vi "Teleop.vi"(10 "Match Info":T1={"Autonomous Elapsed Seconds"=0.0, "TeleOp Elapsed Seconds"=0.0, "Disabled Elapsed Seconds"=0.0, "Visited Autonomous"=FALSE, "Visited TeleOp"=FALSE, "Visited Disabled"=FALSE, "Autonomous Settings"={"Autonomous Style"=enum."Independent", "VI Refnum"=refnum}}, 11 "Call Context":T2) -> ()   [LabVIEW 2019]
doc: "This VI is called for each TeleOp packet received from the DS where the robot is not disabled. It is often used to read from the joysticks and update I/O or to update setpoints for timed control loops. It should complete and return within 20 milliseconds or it may miss DS packets."
uses:
  <vilib>/Rock Robotics/WPI/DriverStation/WPI_DriverStationDerivedRobotMode.ctl
  <vilib>/Rock Robotics/WPI/DriverStation/WPI_DriverStationMatch Info.ctl
  <vilib>/Rock Robotics/WPI/Utilities/WPI_GetSetVariantRefNum.vi
  <vilib>/Rock Robotics/Network Tables/NT Read Number.vi
  Robot Global Data.vi
  <vilib>/Rock Robotics/Network Tables/NT Write Number.vi
panel:
  # "Click here to set min"
  # "Click here to set max"
  # "Click here to set min"
  # "Click here to set max"
  # "Click here to set min"
  # "Click here to set max"
  # "Click here to set min"
  # "Click here to set max"
  # "Click here to set min"
  # "Click here to set max"
  # "Click here to set min"
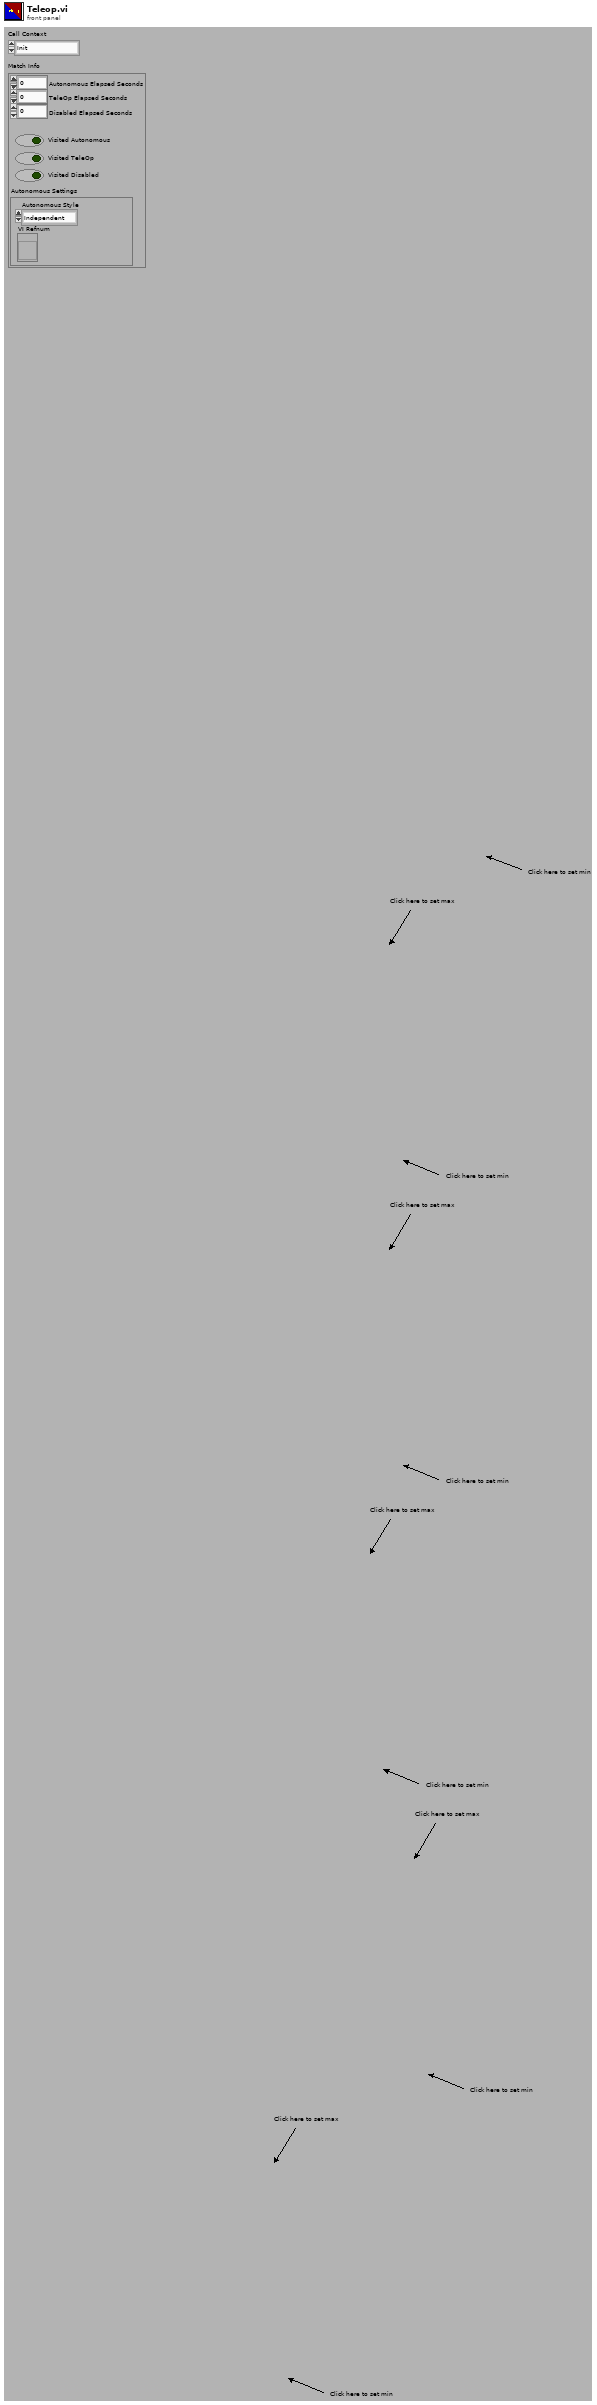
[diagram p1: front panel]
types:
  T1 = typedef "WPI_DriverStationMatch Info.ctl" = cluster{"Autonomous Elapsed Seconds":dbl, "TeleOp Elapsed Seconds":dbl, "Disabled Elapsed Seconds":dbl, "Visited Autonomous":bool, "Visited TeleOp":bool, "Visited Disabled":bool, "Autonomous Settings":cluster{"Autonomous Style":enum16{"Iterative", "Independent"}, "VI Refnum":refnum<vi>}}
  T2 = typedef "WPI_DriverStationDerivedRobotMode.ctl" = enum16{"Init", "Execute", "Stop"}
  T3 = typedef "WPI_MotorControlDeviceRef.ctl" = cluster{"DeviceStatus":errorcluster, "Type":T4, "PWM":cluster{"PWM Channel":T5, "DeadBand":T6}, "CAN":cluster{"Device Number":u8, "SetOutput VI Ref":variant, "GetOutput VI Ref":variant, "Enable VI Ref":variant, "Disable VI Ref":variant, "Data":variant}, "Invert":bool, "DIO PWM":cluster{"PWM \"Enable\" Channel":T5, "DIOChannel":T7, "PWM Rate":dbl}}
  T4 = typedef "WPI_MotorControlType.ctl" = enum16{"PWM", "CAN", "DIO PWM"}
  T5 = typedef "FPGA_DIOPWMChannel.ctl" = enum8{"PWM 0", "PWM 1", "PWM 2", "PWM 3", "PWM 4", "PWM 5", "PWM 6", "PWM 7", "PWM 8", "PWM 9", "PWM MXP 0", "PWM MXP 1", "PWM MXP 2", "PWM MXP 3", "PWM MXP 4", "PWM MXP 5", "PWM MXP 6", "PWM MXP 7", "PWM MXP 8", "PWM MXP 9", "Invalid"}
  T6 = typedef "WPI_PWMDeadband.ctl" = cluster{"Name":string, "maxPositivePwm":i32, "minPositivePwm":i32, "centerPwm":i32, "maxNegativePwm":i32, "minNegativePwm":i32, "angularRange":u16}
  T7 = typedef "FPGA_DIOChannel.ctl" = enum8{"DIO 0", "DIO 1", "DIO 2", "DIO 3", "DIO 4", "DIO 5", "DIO 6", "DIO 7", "DIO 8", "DIO 9", "DIO MXP 0", "DIO MXP 1", "DIO MXP 2", "DIO MXP 3", "DIO MXP 4", "DIO MXP 5", "DIO MXP 6", "DIO MXP 7", "DIO MXP 8", "DIO MXP 9", "DIO MXP 10", "DIO MXP 11", "DIO MXP 12", "DIO MXP 13", "DIO MXP 14", "DIO MXP 15", "SPI Port CS1", "SPI Port CS2", "SPI Port CS3", "SPI Port MISO", "SPI Port MOSI", "Invalid"}
  T8 = typedef "WPI_JoystickDevRef.ctl" = cluster{"Device":T9}
  T9 = typedef "WPI_JoystickDeviceEnum.ctl" = enum16{"USB 0", "USB 1", "USB 2", "USB 3", "USB 4", "USB 5"}
  T10 = typedef "WPI_RobotDriveDevRef.ctl" = cluster{"DevStatus":errorcluster, "Motors[]":T3[], "Square Inputs":bool, "Max Output":dbl}
  T11 = cluster{"JoystickDevRef":T8, "RobotDriveDevRef":T10}
  T12 = typedef "WPI_ServoDeviceRef.ctl" = cluster{"DeviceStatus":errorcluster, "PWM Channel":T5, "DeadBand":T6}
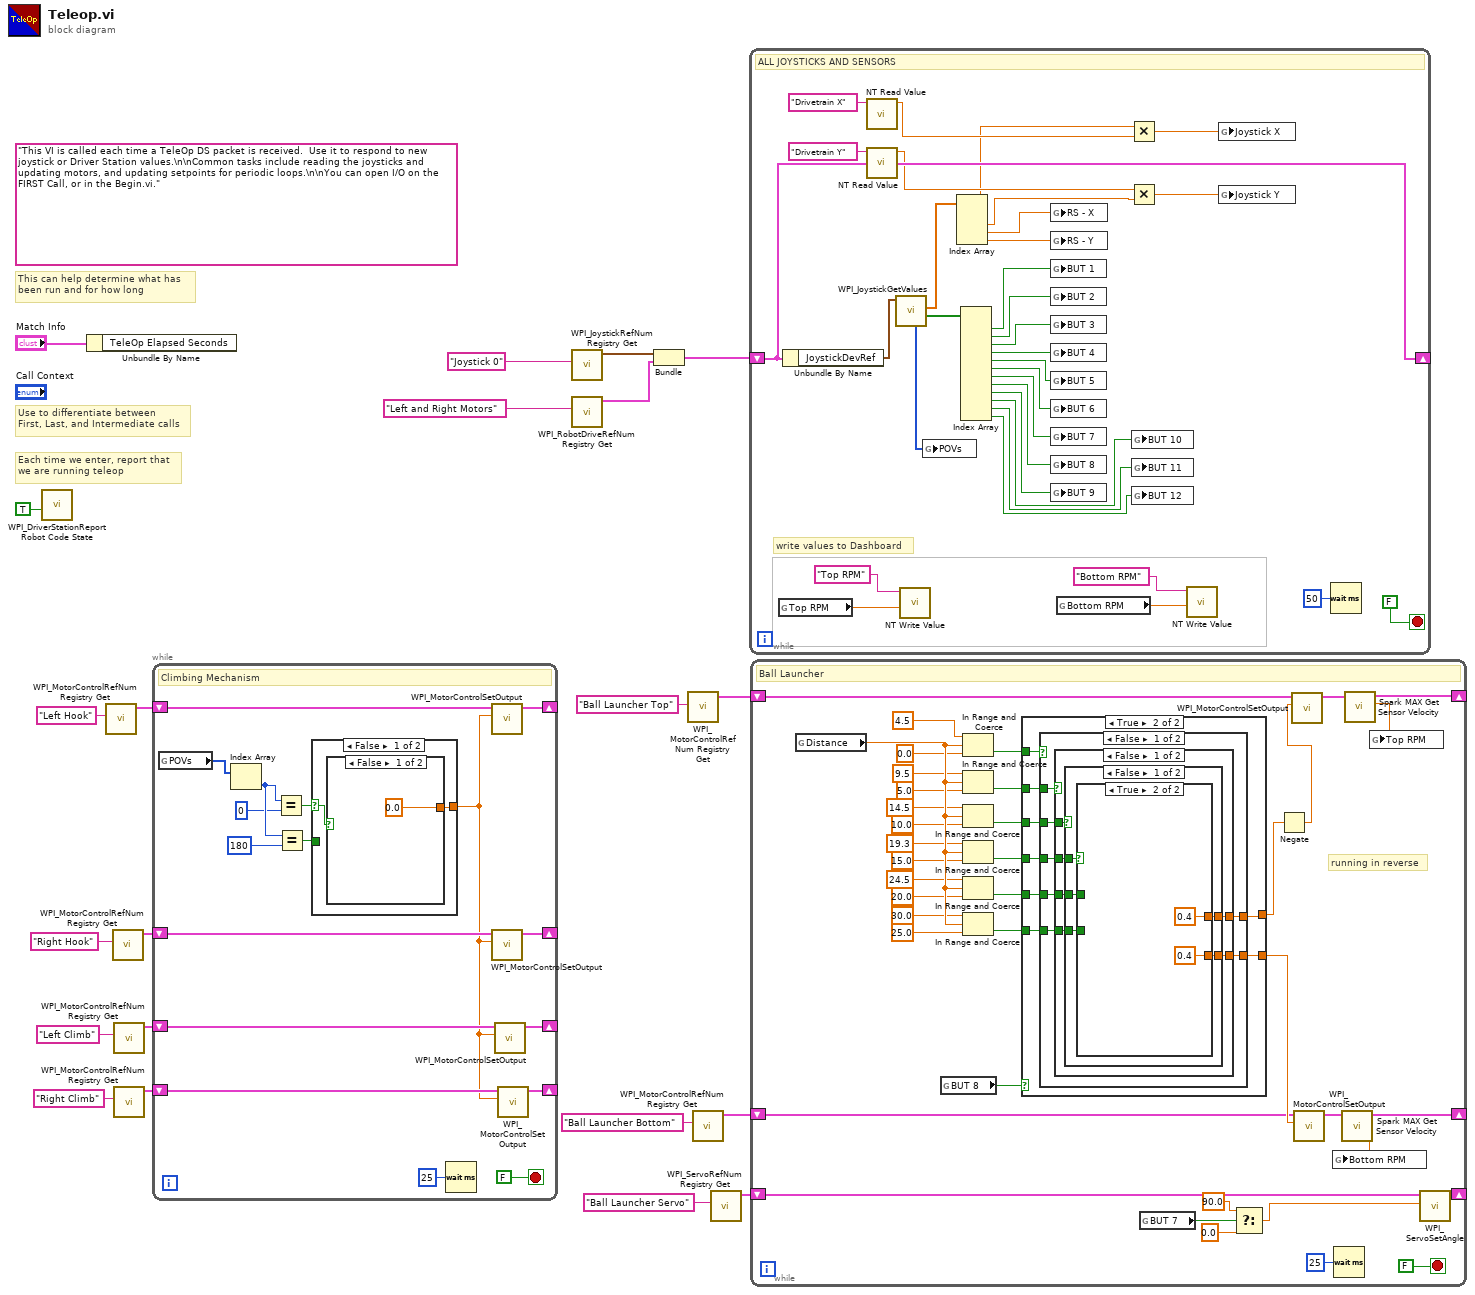
[diagram p0: block diagram]
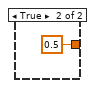
[diagram p2: hidden frame]
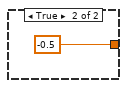
[diagram p3: hidden frame]
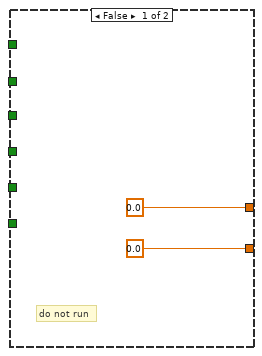
[diagram p4: hidden frame]
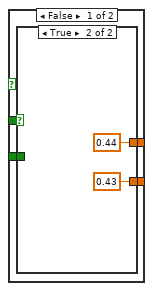
[diagram p5: hidden frame]
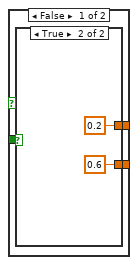
[diagram p6: hidden frame]
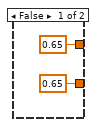
[diagram p7: hidden frame]
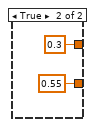
[diagram p8: hidden frame]
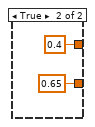
[diagram p9: hidden frame]
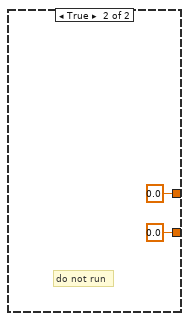
[diagram p10: hidden frame]
diagram:
  (unwired) "This VI is called each time a TeleOp DS packet is received.  Use it to respond to new joystick or Driver Station values.\n\nCommon tasks include reading the joysticks and updating motors, and updating setpoints for periodic loops.\n\nYou can open I/O on the FIRST Call, or in the Begin.vi."
  # "Each time we enter, report that\nwe are running teleop"
  # "Use to differentiate between\nFirst, Last, and Intermediate calls"
  # "This can help determine what has\nbeen run and for how long"
  n1 = call <vilib>:"WPI_DriverStationReport Robot Code State.vi"("TeleOp"=TRUE ("Autonomous")) -> ()  [unwired: 10 in, 1 out]
  n2 = Unbundle By Name("Match Info") -> ()  [unwired: 1 out]
  n3 = call <vilib>:"WPI_MotorControlRefNum Registry Get.vi"("refnum name"="Left Hook") -> ("MotorControlDevRef"=w10:T3)  [unwired: 9 in, 1 out]
  n4 = call <vilib>:"WPI_MotorControlRefNum Registry Get.vi"("refnum name"="Right Hook") -> ("MotorControlDevRef"=w7:T3)  [unwired: 9 in, 1 out]
  n5 = call <vilib>:"WPI_MotorControlRefNum Registry Get.vi"("refnum name"="Left Climb") -> ("MotorControlDevRef"=w3:T3)  [unwired: 9 in, 1 out]
  n6 = call <vilib>:"WPI_MotorControlRefNum Registry Get.vi"("refnum name"="Right Climb") -> ("MotorControlDevRef"=w6:T3)  [unwired: 9 in, 1 out]
  n7 = while {
    shift-right: [w36] -> _
    shift-left: w10 -> [w35]
    shift-right: [w34] -> _
    shift-left: w7 -> [w33]
    shift-right: [w25] -> _
    shift-left: w6 -> [w26]
    shift-right: [w23] -> _
    shift-left: w3 -> [w24]
    stop <- FALSE stop-if-true
    # "Climbing Mechanism"
    n8 = global read "Robot Global Data.vi" "POVs"() -> (w31:i16[])
    n9 = Index Array(array=w31) -> (element=w29:i16)  [unwired: 1 in]
    n10 = Equal?(x=w29, y=i16 0) -> (x = y?=w32:bool)
    n11 = Equal?(x=w29, y=i16 180) -> (x = y?=w30:bool)
    n12 = case shown="False" w32 {
      selector: w32 -> [w39 _]
      tunnel: w30 -> [_ _]
      tunnel: [w40 -0.5 ("Output")] -> w22
      frame False {
        n13 = case shown="False" w39 {
          tunnel: [0.0 ("Output") 0.5 ("Output")] -> w40
          frame False {
          }
          frame True {
          }
        }
      }
      frame True {
      }
    }
    n14 = Wait (ms)(milliseconds to wait=u32 25) -> ()  [unwired: 1 out]
    n15 = call <vilib>:"WPI_MotorControlSetOutput.vi"("Output"=w22, "MotorControlDevRef"=w35) -> ("MotorControlDevRef"=w36:T3)  [unwired: 7 in, 2 out]
    n16 = call <vilib>:"WPI_MotorControlSetOutput.vi"("Output"=w22, "MotorControlDevRef"=w33) -> ("MotorControlDevRef"=w34:T3)  [unwired: 7 in, 2 out]
    n17 = call <vilib>:"WPI_MotorControlSetOutput.vi"("Output"=w22, "MotorControlDevRef"=w24) -> ("MotorControlDevRef"=w23:T3)  [unwired: 7 in, 2 out]
    n18 = call <vilib>:"WPI_MotorControlSetOutput.vi"("Output"=w22, "MotorControlDevRef"=w26) -> ("MotorControlDevRef"=w25:T3)  [unwired: 7 in, 2 out]
  }
  n19 = call <vilib>:"WPI_JoystickRefNum Registry Get.vi"("refnum name"="Joystick 0") -> ("JoystickDevRef"=w17:T8)  [unwired: 1 in, 9 out]
  n20 = call <vilib>:"WPI_RobotDriveRefNum Registry Get.vi"("refnum name"="Left and Right Motors") -> ("RobotDriveDevRef"=w16:T10)  [unwired: 1 in, 9 out]
  n21 = Bundle("JoystickDevRef"=w17, "RobotDriveDevRef"=w16) -> (w15:T11)  [unwired: 1 out]
  n22 = call <vilib>:"WPI_MotorControlRefNum Registry Get.vi"("refnum name"="Ball Launcher Top") -> ("MotorControlDevRef"=w11:T3)  [unwired: 9 in, 1 out]
  n23 = call <vilib>:"WPI_MotorControlRefNum Registry Get.vi"("refnum name"="Ball Launcher Bottom") -> ("MotorControlDevRef"=w13:T3)  [unwired: 9 in, 1 out]
  n24 = call <vilib>:"WPI_ServoRefNum Registry Get.vi"("refnum name"="Ball Launcher Servo") -> ("ServoDeviceRef"=w1:T12)  [unwired: 9 in, 1 out]
  n25 = while {
    shift-right: [w61] -> _
    shift-left: w15 -> [w61]
    stop <- FALSE stop-if-true
    # "write values to Dashboard"
    # "ALL JOYSTICKS AND SENSORS"
    n26 = global read "Robot Global Data.vi" "Top RPM"() -> (w55:dbl)
    n27 = Unbundle By Name(w61) -> ("JoystickDevRef"=w75:T8)
    n28 = call-poly <vilib>:"NT Read Value.vi"("Name"="Drivetrain X") -> ("Numeric"=w49:dbl)  [unwired: 9 in, 1 out]
    n29 = call-poly <vilib>:"NT Read Value.vi"("Name"="Drivetrain Y") -> ("Numeric"=w50:dbl)  [unwired: 9 in, 1 out]
    n30 = call <vilib>:"WPI_JoystickGetValues.vi"("JoystickDevRef"=w75) -> ("Buttons"=w74:bool[], "Axes"=w60:dbl[], "POVs"=w44:i16[])  [unwired: 6 in, 2 out]
    n31 = call-poly <vilib>:"NT Write Value.vi"("Numeric"=w55, "Name"="Top RPM") -> ()  [unwired: 9 in, 1 out]
    n32 = global write "Robot Global Data.vi" "POVs"(w44) -> ()
    n33 = Index Array(array=w60) -> (element #1=w46:dbl, element #2=w45:dbl, element #3=w47:dbl, element #4=w58:dbl)  [unwired: 4 in]
    n34 = Index Array(array=w74) -> (element #1=w73:bool, element #2=w72:bool, element #3=w71:bool, element #4=w70:bool, element #5=w69:bool, element #6=w68:bool, element #7=w67:bool, element #8=w66:bool, element #9=w65:bool, element #10=w64:bool, element #11=w63:bool, element #12=w62:bool)  [unwired: 12 in]
    n35 = global write "Robot Global Data.vi" "RS - X"(w47) -> ()
    n36 = global write "Robot Global Data.vi" "RS - Y"(w58) -> ()
    n37 = global write "Robot Global Data.vi" "BUT 1"(w73) -> ()
    n38 = global write "Robot Global Data.vi" "BUT 2"(w72) -> ()
    n39 = global write "Robot Global Data.vi" "BUT 3"(w71) -> ()
    n40 = global write "Robot Global Data.vi" "BUT 4"(w70) -> ()
    n41 = global write "Robot Global Data.vi" "BUT 5"(w69) -> ()
    n42 = global write "Robot Global Data.vi" "BUT 6"(w68) -> ()
    n43 = global write "Robot Global Data.vi" "BUT 7"(w67) -> ()
    n44 = global write "Robot Global Data.vi" "BUT 8"(w66) -> ()
    n45 = global write "Robot Global Data.vi" "BUT 9"(w65) -> ()
    n46 = global read "Robot Global Data.vi" "Bottom RPM"() -> (w53:dbl)
    n47 = Multiply(x=w46, y=w49) -> (x*y=w48:dbl)
    n48 = Multiply(x=w50, y=w45) -> (x*y=w59:dbl)
    n49 = global write "Robot Global Data.vi" "BUT 10"(w64) -> ()
    n50 = global write "Robot Global Data.vi" "BUT 11"(w63) -> ()
    n51 = global write "Robot Global Data.vi" "BUT 12"(w62) -> ()
    n52 = call-poly <vilib>:"NT Write Value.vi"("Numeric"=w53, "Name"="Bottom RPM") -> ()  [unwired: 9 in, 1 out]
    n53 = global write "Robot Global Data.vi" "Joystick X"(w48) -> ()
    n54 = global write "Robot Global Data.vi" "Joystick Y"(w59) -> ()
    n55 = Wait (ms)(milliseconds to wait=u32 50) -> ()  [unwired: 1 out]
  }
  n56 = while {
    shift-right: [w85] -> _
    shift-left: w13 -> [w86]
    shift-right: [w83] -> _
    shift-left: w11 -> [w84]
    shift-right: [w82] -> _
    shift-left: w1 -> [w77]
    stop <- FALSE stop-if-true
    # "running in reverse"
    # "Ball Launcher"
    n57 = global read "Robot Global Data.vi" "Distance"() -> (w115:dbl)
    n58 = global read "Robot Global Data.vi" "BUT 8"() -> (w93:bool)
    n59 = In Range and Coerce(upper limit=4.5, x=w115, lower limit=0.0) -> (In Range?=w112:bool)  [unwired: 1 out]
    n60 = In Range and Coerce(upper limit=9.5, x=w115, lower limit=5.0) -> (In Range?=w111:bool)  [unwired: 1 out]
    n61 = In Range and Coerce(upper limit=14.5, x=w115, lower limit=10.0) -> (In Range?=w95:bool)  [unwired: 1 out]
    n62 = In Range and Coerce(upper limit=19.3, x=w115, lower limit=15.0) -> (In Range?=w96:bool)  [unwired: 1 out]
    n63 = In Range and Coerce(upper limit=24.5, x=w115, lower limit=20.0) -> (In Range?=w97:bool)  [unwired: 1 out]
    n64 = In Range and Coerce(upper limit=30.0, x=w115, lower limit=25.0) -> (In Range?=w98:bool)  [unwired: 1 out]
    n65 = case shown="True" w93 {
      tunnel: [0.0 ("Output") w119] -> w114
      tunnel: [0.0 ("Output") w118] -> w94
      tunnel: w112 -> [_ w125]
      tunnel: w95 -> [_ w123]
      tunnel: w96 -> [_ w122]
      tunnel: w97 -> [_ w121]
      tunnel: w98 -> [_ w120]
      tunnel: w111 -> [_ w124]
      frame False {
        # "do not run"
      }
      frame True {
        n66 = case shown="False" w125 {
          tunnel: w124 -> [w132 _]
          tunnel: w123 -> [w131 _]
          tunnel: w122 -> [w130 _]
          tunnel: w121 -> [w129 _]
          tunnel: w120 -> [w128 _]
          tunnel: [w127 0.0 ("Output")] -> w119
          tunnel: [w126 0.0 ("Output")] -> w118
          frame False {
            n67 = case shown="False" w132 {
              tunnel: w131 -> [w138 _]
              tunnel: w130 -> [w137 _]
              tunnel: w129 -> [w136 _]
              tunnel: w128 -> [w135 _]
              tunnel: [w134 0.4 ("Output")] -> w127
              tunnel: [w133 0.65 ("Output")] -> w126
              frame False {
                n68 = case shown="False" w138 {
                  tunnel: w137 -> [w143 _]
                  tunnel: w136 -> [w142 _]
                  tunnel: w135 -> [w141 _]
                  tunnel: [w140 0.3 ("Output")] -> w134
                  tunnel: [w139 0.55 ("Output")] -> w133
                  frame False {
                    n69 = case shown="True" w143 {
                      tunnel: w142 -> [w147 _]
                      tunnel: w141 -> [w146 _]
                      tunnel: [w145 0.4 ("Output")] -> w140
                      tunnel: [w144 0.4 ("Output")] -> w139
                      frame False {
                        n70 = case shown="True" w147 {
                          tunnel: w146 -> [w150 _]
                          tunnel: [w149 0.44 ("Output")] -> w145
                          tunnel: [w148 0.43 ("Output")] -> w144
                          frame False {
                            n71 = case shown="True" w150 {
                              tunnel: [0.65 ("Output") 0.2 ("Output")] -> w149
                              tunnel: [0.65 ("Output") 0.6 ("Output")] -> w148
                              frame False {
                              }
                              frame True {
                              }
                            }
                          }
                          frame True {
                          }
                        }
                      }
                      frame True {
                      }
                    }
                  }
                  frame True {
                  }
                }
              }
              frame True {
              }
            }
          }
          frame True {
            # "do not run"
          }
        }
      }
    }
    n72 = global read "Robot Global Data.vi" "BUT 7"() -> (w81:bool)
    n73 = Select(t=90.0, s=w81, f=0.0) -> (s? t:f=w78:dbl)
    n74 = Negate(x=w114) -> (-x=w113:dbl)
    n75 = call <vilib>:"WPI_MotorControlSetOutput.vi"("Output"=w113, "MotorControlDevRef"=w84) -> ("MotorControlDevRef"=w91:T3)  [unwired: 7 in, 2 out]
    n76 = call <vilib>:"WPI_MotorControlSetOutput.vi"("Output"=w94, "MotorControlDevRef"=w86) -> ("MotorControlDevRef"=w92:T3)  [unwired: 7 in, 2 out]
    n77 = Wait (ms)(milliseconds to wait=u32 25) -> ()  [unwired: 1 out]
    n78 = call <vilib>:"Spark MAX Get Sensor Velocity.vi"("MotorControlDevRef in"=w92) -> ("Sensor Velocity"=w90:dbl, "MotorControlDevRef out"=w85:T3)  [unwired: 7 in, 2 out]
    n79 = global write "Robot Global Data.vi" "Bottom RPM"(w90) -> ()
    n80 = call <vilib>:"Spark MAX Get Sensor Velocity.vi"("MotorControlDevRef in"=w91) -> ("Sensor Velocity"=w89:dbl, "MotorControlDevRef out"=w83:T3)  [unwired: 7 in, 2 out]
    n81 = global write "Robot Global Data.vi" "Top RPM"(w89) -> ()
    n82 = call <vilib>:"WPI_ServoSetAngle.vi"("Angle"=w78, "ServoDeviceRef"=w77) -> ("ServoDeviceRef"=w82:T12)  [unwired: 8 in, 1 out]
  }
